vi "Measure.vi"(0 "Keysight_34401A-DMM in":refnum<class "Keysight_34401A-DMM.lvclass">, 11 "error in (no error)":errorcluster) -> (4 "Keysight_34401A-DMM out":refnum<class "Keysight_34401A-DMM.lvclass">, 6 "Measure_Results":variant, 15 "error out":errorcluster)   [LabVIEW 2020, in "AbstractDMM.lvlib" / "Keysight_34401A-DMM.lvclass"]
uses:
  Keysight_34401A-DMM.lvclass
  Keysight_34401A-DMM.lvclass/Keysight_34401A-DMM.ctl
  <instrlib>/Agilent 34401/Public/Data/Read (Single Point).vi
  <instrlib>/Agilent 34401/Agilent 34401.lvlib
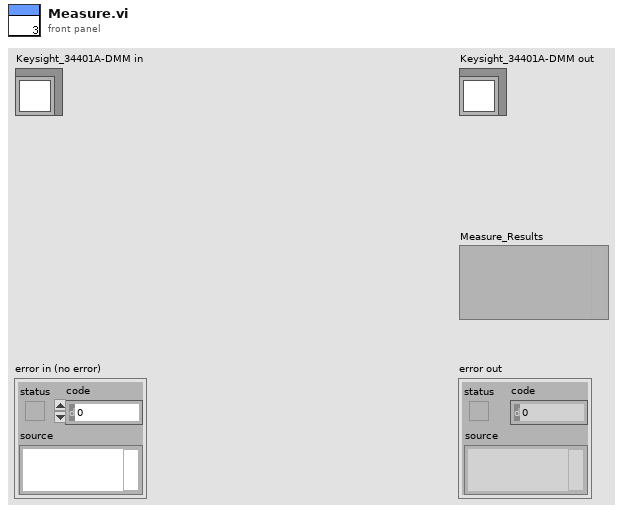
[diagram p1: front panel]
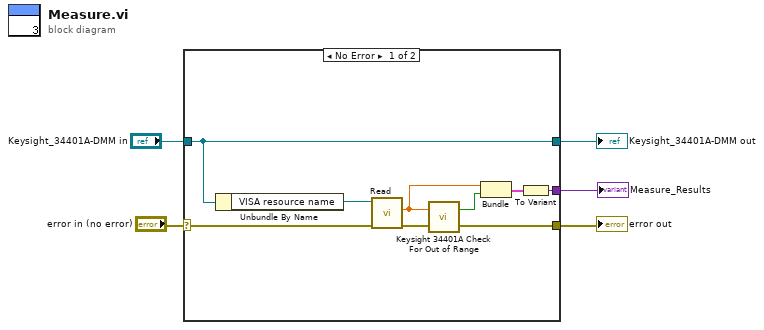
[diagram p0: block diagram]
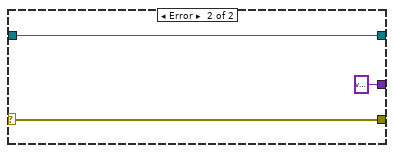
[diagram p2: hidden frame]
diagram:
  n1 = case shown="No Error" "error in (no error)" {
    selector: "error in (no error)" -> [w13 w14]
    tunnel: [w12 w14] -> w4
    tunnel: "Keysight_34401A-DMM in" -> [w6 w16]
    tunnel: [w7 variant ("Variant")] -> w2
    tunnel: [w6 w16] -> w1
    frame No Error {
      n2 = Unbundle By Name(w6) -> ("VISA resource name"=w11:refnum<visa-resource-name>)
      n3 = call-poly <instrlib>:"Read.vi"("error in (no error)"=w13, "VISA resource name"=w11) -> ("error out"=w12:errorcluster, "Measurement"=w10:dbl)  [unwired: 7 in, 1 out]
      n4 = call "Keysight 34401A Check For Out of Range.vi"("value"=w10) -> ("out of range?"=w9:bool)  [unwired: 2 in]
      n5 = Bundle("Measurement"=w10, "out of range?"=w9) -> (w8:cluster{"Measurement":dbl, "out of range?":bool})  [unwired: 1 in]
      n6 = To Variant(anything=w8) -> (Variant=w7:variant)
    }
    frame Error {
    }
  }
  "error out" <- w4
  "Keysight_34401A-DMM out" <- w1
  "Measure_Results" <- w2
